vi "Radar.vi"() -> ()   [LabVIEW 2020]
panel:
  in  "Enter Numeric Value For Activate":string
  out "Ultrasonic distance":dbl
  in  "byte Ultrsonic":u32
  out "Servo Rotation":string
  in  "byte Servo":u32
  in  "VISA resource name":refnum<visa-resource-name>
  in  "stop":bool
  out "Radar Project":picture
  # "LabVIEW + Arduino + Radar Project"
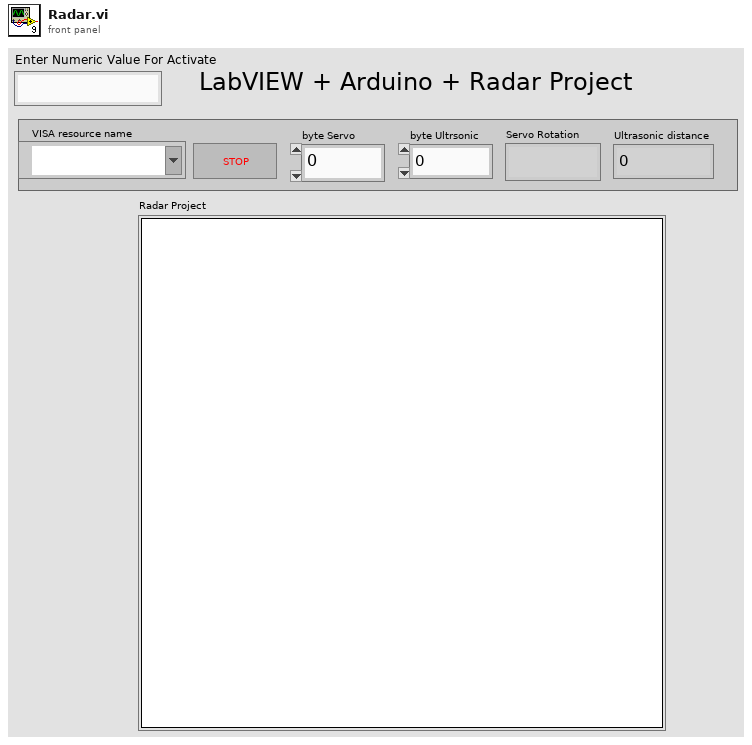
[diagram p1: front panel]
types:
  T1 = cluster{"maximum":dbl, "minimum":dbl, "clip to min":bool, "log?(F)":bool, "grid color":u32, "plot color":u32, "fmt and prec":cluster{"format":enum8{"Decimal", "Scientific", "Engineering", "Binary", "Octal", "Hex"}, "precision":u8}, "visible section":u16}
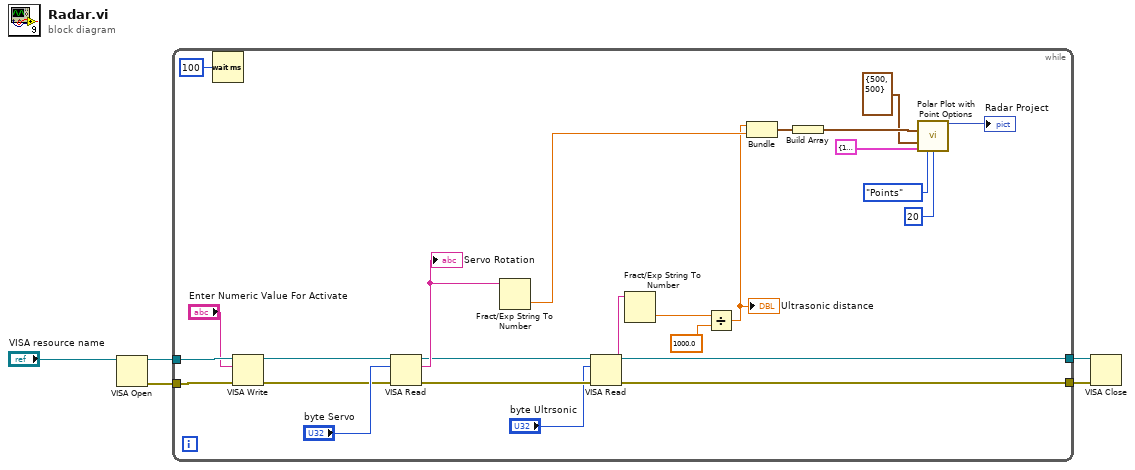
[diagram p0: block diagram]
diagram:
  n1 = VISA Open(VISA resource name="VISA resource name") -> (VISA resource name=w5:refnum<visa-resource-name>, error out=w4:errorcluster)  [unwired: 4 in]
  n2 = while {
    tunnel: w5 -> [w10]
    tunnel: w4 -> [w9]
    tunnel: [w18] -> w2
    tunnel: [w17] -> w1
    stop <- "stop" stop-if-true
    n3 = Wait (ms)(milliseconds to wait=u32 100) -> ()  [unwired: 1 out]
    n4 = VISA Write(VISA resource name=w10, write buffer="Enter Numeric Value For Activate", error in (no error)=w9) -> (VISA resource name out=w8:refnum<visa-resource-name>, error out=w7:errorcluster)  [unwired: 1 out]
    n5 = VISA Read(VISA resource name=w8, byte count="byte Servo", error in (no error)=w7) -> (VISA resource name out=w20:refnum<visa-resource-name>, read buffer=w22:string, error out=w19:errorcluster)  [unwired: 1 out]
    "Servo Rotation" <- w22
    n6 = Fract/Exp String To Number(string=w22) -> (number=w21:dbl)  [unwired: 3 in, 1 out]
    n7 = VISA Read(VISA resource name=w20, byte count="byte Ultrsonic", error in (no error)=w19) -> (VISA resource name out=w18:refnum<visa-resource-name>, read buffer=w15:string, error out=w17:errorcluster)  [unwired: 1 out]
    n8 = Fract/Exp String To Number(string=w15) -> (number=w12:dbl)  [unwired: 3 in, 1 out]
    n9 = Divide(x=w12, y=1000.0) -> (x/y=w11:dbl)
    "Ultrasonic distance" <- w11
    n10 = Bundle "Bundle"(w11, w21) -> (w31:cluster{dbl, dbl})  [unwired: 1 in]
    n11 = Build Array "Build Array"(w31) -> (w30:cluster{dbl, dbl}[])
    n12 = call <vilib>:"Polar Plot with Point Options.vi"("data array [mag, phase (deg)]"=w30, "dimensions (w,h)"=cluster{"width":i16, "height":i16} {"width"=500, "height"=500}, "polar attributes"=T1 {"maximum"=10.0, "minimum"=0.0, "clip to min"=FALSE, "log?(F)"=FALSE, "grid color"=16860, "plot color"=16711680, "fmt and prec"={"format"=enum."Decimal", "precision"=2}, "visible section"=8}, "Lines/Points"=enum16{"Lines", "Points"}."Points", "Size"=u16 20) -> ("new picture"=→"Radar Project":picture)  [unwired: 10 in]
  }
  n13 = VISA Close(VISA resource name=w2, error in (no error)=w1) -> ()  [unwired: 1 out]
